vi "Send Channel Data.vi"(8 "Max3":u32, 9 "Max2":u32, 10 "Max1":u32, 11 "Max0":u32) -> ()   [LabVIEW 2017]
uses:
  <vilib>/rvi/DataTransferAndStorage/Container/XNode/niFpgaContainer.xnode
  <vilib>/rvi/Memory/Memory_Emulation/nirvimemoryEmulation.vi
  <vilib>/rvi/Memory/Memory_Emulation/nirvimemoryFastEmulation.vi
  <vilib>/rvi/FXPMathLib/FxpAdd/XNode/nifxpmath_Add.xnode
  <vilib>/rvi/FXPMathLib/sim/FxpSim.dll
  <vilib>/rvi/DataTransferAndStorage/Register/Emulation/niFpgaRegisterEmulation.vi
  <vilib>/rvi/interface/RandomDataEmulation/nirviRandomDataFpgaReadWriteTemplate.vi
  <vilib>/rvi/FIFO/Fifo_Resource/niFpgaFifoEmulationRefIn.vi
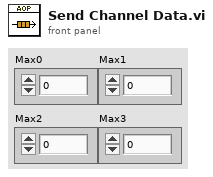
[diagram p1: front panel]
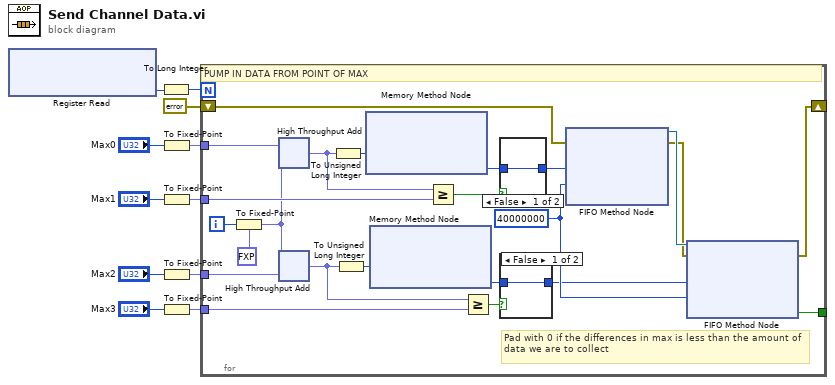
[diagram p0: block diagram]
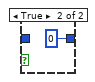
[diagram p2: hidden frame]
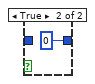
[diagram p3: hidden frame]
diagram:
  n1 = xnode ("Register Read")() -> ("Data"=w8:u16)  [unwired: 1 in, 1 out]
  n2 = To Long Integer(number=w8) -> (32bit integer=w9:i32)
  n3 = To Fixed-Point(number="Max0") -> (fixed-point=w11:fxp<+,32,32>)  [unwired: 1 in]
  n4 = To Fixed-Point(number="Max1") -> (fixed-point=w7:fxp<+,32,32>)  [unwired: 1 in]
  n5 = To Fixed-Point(number="Max2") -> (fixed-point=w10:fxp<+,32,32>)  [unwired: 1 in]
  n6 = To Fixed-Point(number="Max3") -> (fixed-point=w6:fxp<+,32,32>)  [unwired: 1 in]
  n7 = for {
    N: w9 -> [_]
    tunnel: [w31] -> _
    tunnel: w7 -> [w29]
    tunnel: w11 -> [w22]
    tunnel: w10 -> [w17]
    tunnel: w6 -> [w18]
    shift-right: [w13] -> _
    shift-left: errorcluster {"Status?"=FALSE, "Code"=0, "Source"=""} ("error out") -> [w12]
    i -> [w20]
    w32 = 40000000 ("Timeout")
    # "Pad with 0 if the differences in max is less than the amount of data we are to collect"
    # "PUMP IN DATA FROM POINT OF MAX"
    n8 = To Fixed-Point(fixed-point type=fxp<+,32,32> 0.0, number=w20) -> (fixed-point=w21:fxp<+,32,32>)
    n9 = xnode ("High Throughput Add")("x"=w22, "y"=w21) -> ("x+y"=w19:fxp<+,32,32>)
    n10 = xnode ("High Throughput Add")("x"=w21, "y"=w17) -> ("x+y"=w16:fxp<+,32,32>)
    n11 = To Unsigned Long Integer(number=w19) -> (unsigned 32bit integer=w34:u32)
    n12 = To Unsigned Long Integer(number=w16) -> (unsigned 32bit integer=w30:u32)
    n13 = xnode ("Memory Method Node")("Address"=w34) -> ("Data"=w27:i16)  [unwired: 1 in, 1 out]
    n14 = xnode ("Memory Method Node")("Address"=w30) -> ("Data"=w24:i16)  [unwired: 1 in, 1 out]
    n15 = Greater Or Equal?(x=w19, y=w29) -> (x >= y?=w28:bool)
    n16 = Greater Or Equal?(x=w16, y=w18) -> (x >= y?=w25:bool)
    n17 = case shown="False" w28 {
      tunnel: w27 -> [w37 _]
      tunnel: [w37 i16 0 ("Data")] -> w26
      frame False {
      }
      frame True {
      }
    }
    n18 = case shown="False" w25 {
      tunnel: w24 -> [w35 _]
      tunnel: [w35 i16 0 ("Data")] -> w23
      frame False {
      }
      frame True {
      }
    }
    n19 = xnode ("FIFO Method Node")("Element"=w26, "Timeout"=w32, "error in (no error)"=w12) -> ("error out"=w14:errorcluster, "FIFO Out"=w33:refnum<k21>)  [unwired: 1 in, 1 out]
    n20 = xnode ("FIFO Method Node")("Element"=w23, "Timeout"=w32, "error in (no error)"=w14, "FIFO In"=w33) -> ("Timed Out?"=w31:bool, "error out"=w13:errorcluster)  [unwired: 1 out]
  }
